vi "Motor_DC_simulado.vi"(6 "Initialize":bool, 7 "dt":dbl=0.01 format="%#_13g", 8 "Velocidade anterior":dbl, 9 "Posiçao anterior":dbl, 10 "DC_Vin":dbl) -> (0 "Tensão fornecida ao motor":dbl, 1 "Aceleração":dbl, 2 "Velocidade":dbl, 3 "Posição":dbl format="%0.2f")   [LabVIEW 2018]
uses:
  <vilib>/ptbypt/NI_PtbyPt.lvlib
  <vilib>/Analysis/NI_AALPro.lvlib
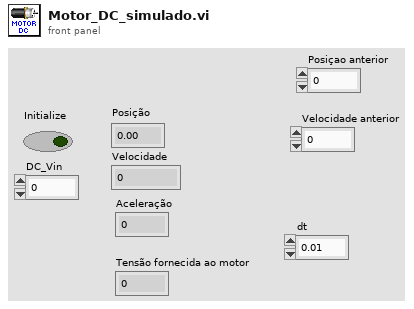
[diagram p1: front panel]
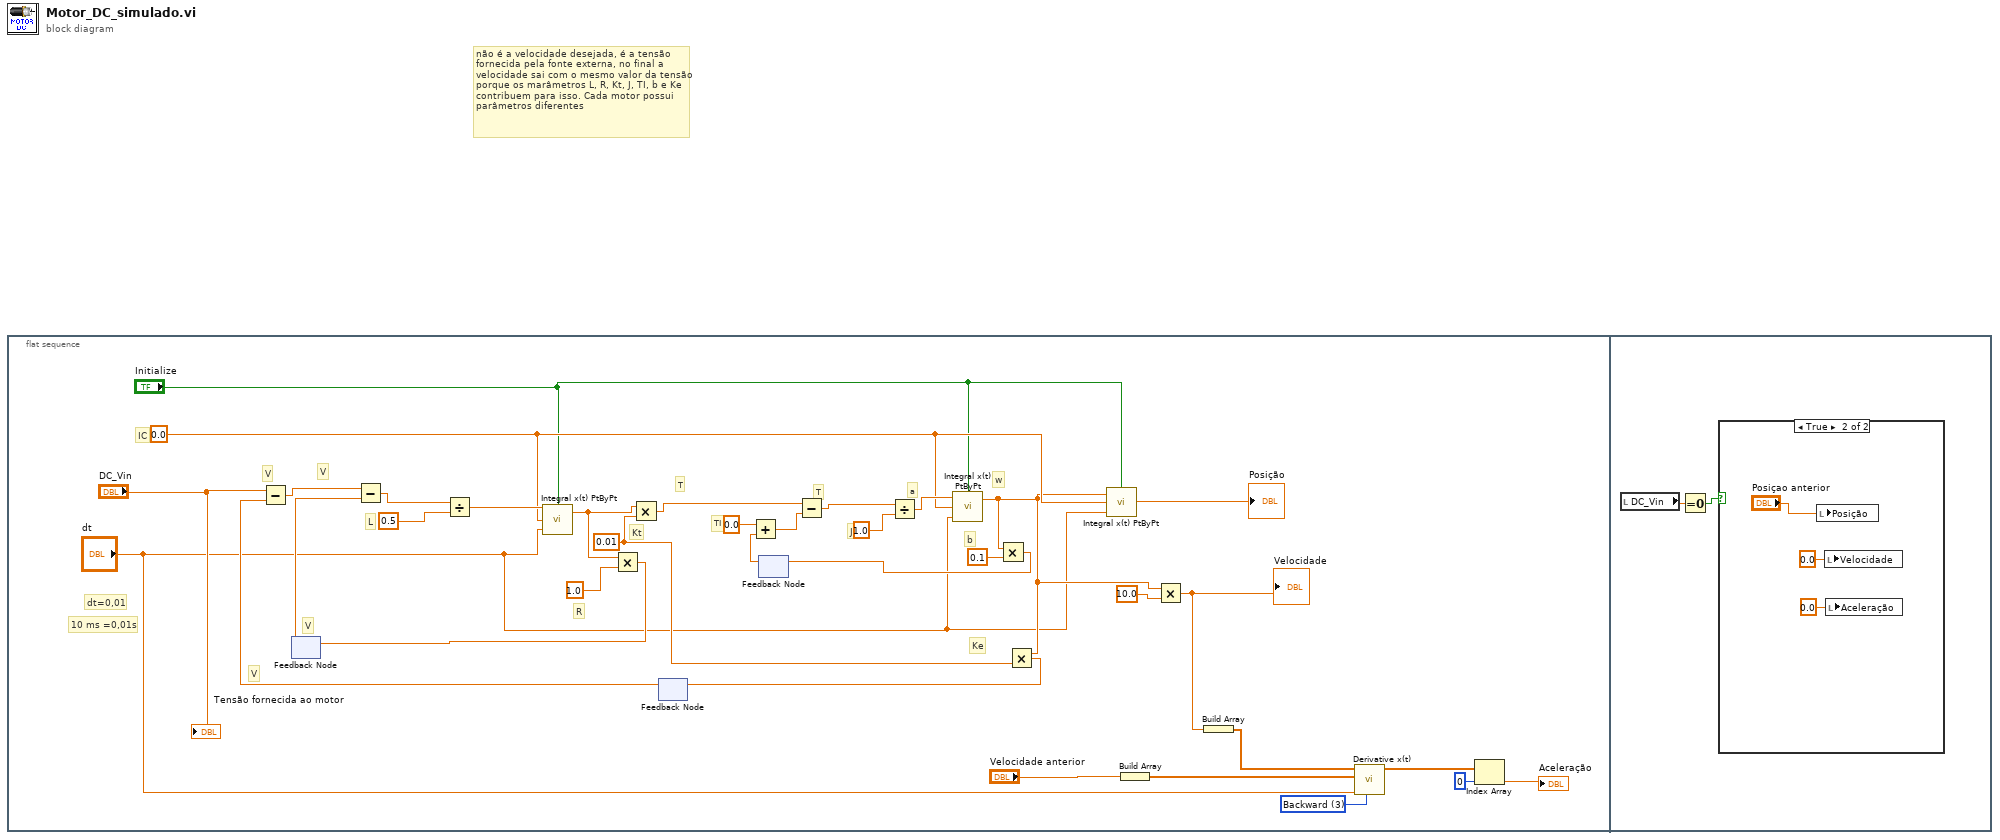
[diagram p0: block diagram]
diagram:
  # "não é a velocidade desejada, é a tensão fornecida pela fonte externa, no final a velocidade sai com o mesmo valor da tensão porque os marâmetros L, R, Kt, J, TI, b e Ke contribuem para isso. Cada motor possui parâmetros diferentes"
  n1 = flat-sequence {
    frame #0 {
      w6 = u16 3 items=["2nd Order Central", "4th Order Central", "Forward", "Backward"] ("method")
      w21 = 0.01 ("y")
      w23 = 0.0
      # "10 ms =0,01s"
      # "dt=0,01"
      # "V"
      # "V"
      # "b"
      # "V"
      # "Ke"
      # "T"
      # "a"
      # "w"
      # "J"
      # "TI"
      # "T"
      # "Kt"
      # "R"
      # "IC"
      # "L"
      # "V"
      n2 = feedback #1() -> (w18:dbl)  [unwired: 1 in]
      n3 = feedback #2() -> (w17:dbl)  [unwired: 1 in]
      n4 = Subtract(x="DC_Vin", y=w17) -> (x-y=w35:dbl)
      n5 = Subtract(x=w35, y=w18) -> (x-y=w34:dbl)
      n6 = Divide(x=w34, y=0.5) -> (x/y=w32:dbl)
      n7 = call <vilib>:"Integral x(t) PtByPt.vi"("initialize"="Initialize", "dt"="dt", "initial condition"=w23, "x"=w32) -> ("integral x(t)"=w31:dbl)  [unwired: 1 out]
      n8 = Multiply(x=w31, y=1.0) -> (x*y=w19:dbl)
      n9 = feedback-in #1(w19) -> ()
      n10 = Multiply(x=w31, y=w21) -> (x*y=w29:dbl)
      n11 = feedback #3() -> (w15:dbl)  [unwired: 1 in]
      n12 = Add(x=0.0, y=w15) -> (x+y=w28:dbl)
      n13 = Subtract(x=w29, y=w28) -> (x-y=w26:dbl)
      n14 = Divide(x=w26, y=1.0) -> (x/y=w24:dbl)
      n15 = call <vilib>:"Integral x(t) PtByPt.vi"("initialize"="Initialize", "dt"="dt", "initial condition"=w23, "x"=w24) -> ("integral x(t)"=w14:dbl)  [unwired: 1 out]
      n16 = Multiply(x=w14, y=0.1) -> (x*y=w12:dbl)
      n17 = feedback-in #3(w12) -> ()
      n18 = Multiply(x=w14, y=w21) -> (x*y=w16:dbl)
      n19 = feedback-in #2(w16) -> ()
      n20 = call <vilib>:"Integral x(t) PtByPt.vi"("initialize"="Initialize", "dt"="dt", "initial condition"=w23, "x"=w14) -> ("integral x(t)"=→"Posição":dbl)  [unwired: 1 out]
      n21 = Build Array("Velocidade anterior") -> (w4:dbl[])
      n22 = Multiply(x=w14, y=10.0) -> (x*y=w8:dbl)
      "Velocidade" <- w8
      n23 = Build Array(w8) -> (w7:dbl[])
      n24 = call <vilib>:"Derivative x(t).vi"("method"=w6, "dt"="dt", "Initial Condition"=w4, "X"=w7) -> ("dX/dt"=w3:dbl[])  [unwired: 6 in, 1 out]
      n25 = Index Array(array=w3, index=0) -> (element=→"Aceleração":dbl)
      "Tensão fornecida ao motor" <- "DC_Vin"
    }
    frame #1 {
      n26 = local read "DC_Vin"() -> (w37:dbl)
      n27 = Equal To 0?(x=w37) -> (x = 0?=w36:bool)
      n28 = case shown="True" w36 {
        frame False {
        }
        frame True {
          n29 = local write "Posição"("Posiçao anterior") -> ()
          n30 = local write "Velocidade"(0.0 ("Velocidade")) -> ()
          n31 = local write "Aceleração"(0.0 ("Aceleração")) -> ()
        }
      }
    }
  }
